vi "Configure StartVelocity Core.vi"(8 "error in (no error)":errorcluster, 9 "StartVelocity":dbl, 10 "AxisNumber":u8, 11 "CS++Nanotec in":refnum<class "CS++Nanotec.lvclass">) -> (0 "error out":errorcluster, 3 "CS++Nanotec out":refnum<class "CS++Nanotec.lvclass">)   [LabVIEW 2015, in "CS++Nanotec.lvlib" / "CS++Nanotec.lvclass"]
doc: "Configures the start (minimum) velocity of the axis."
uses:
  CS++Nanotec.lvclass
  CS++Nanotec.lvclass/CS++Nanotec.ctl
  instr.lib/NanotecSMCPD/NanotecSMCPDDriver.lvlib
  CSPP_DeviceBase/CS++Motor/CS++Motor.lvclass
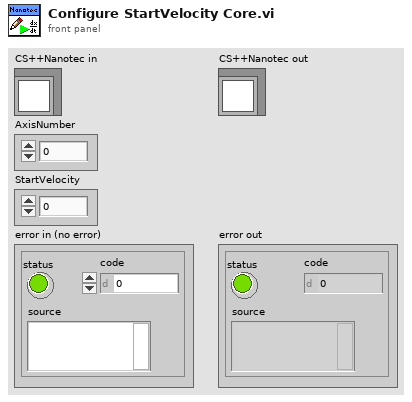
[diagram p1: front panel]
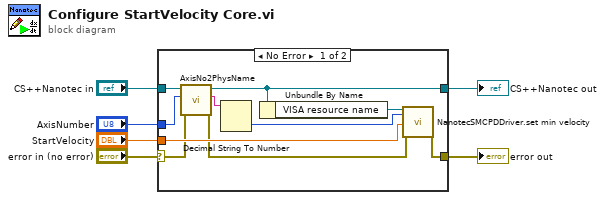
[diagram p0: block diagram]
diagram:
  n1 = case shown="No Error" "error in (no error)" {
    selector: "error in (no error)" -> [w9 w17]
    tunnel: "CS++Nanotec in" -> [w12 w18]
    tunnel: "AxisNumber" -> [w10 _]
    tunnel: "StartVelocity" -> [w15 _]
    tunnel: [w14 w17] -> w2
    tunnel: [w11 w18] -> w1
    frame No Error {
      n2 = call "AxisNo2PhysName.vi"("error in (no error)"=w9, "AxisNumber"=w10, "CS++Motor in"=w12) -> ("error out"=w8:errorcluster, "PhysicalChannelName"=w13:string, "CS++Motor out"=w11:refnum<class "CS++Nanotec.lvclass">)  [unwired: 6 in]
      n3 = Decimal String To Number(string=w13) -> (number=w7:i32)  [unwired: 2 in, 1 out]
      n4 = Unbundle By Name(w11) -> ("VISA resource name"=w16:refnum<visa-resource-name>)
      n5 = call "NanotecSMCPDDriver.set min velocity.vi"("VISA resource name"=w16, "contollerID"=w7, "minVelocity [Hz]"=w15, "error in (no error)"=w8) -> ("error out"=w14:errorcluster)  [unwired: 13 in, 2 out]
    }
    frame Error {
    }
  }
  "error out" <- w2
  "CS++Nanotec out" <- w1
